vi "Configure Transducer.vi"(0 "VISA resource name":refnum<visa-resource-name>, 1 "Thermocouple Type (0: J)":i32(ring) items=["J", "K", "T", "E", "N", "R"], 2 "Enable Thermocouple Check (F: Disable)":bool, 3 "Reference Junction Temperature (0 Degrees C)":dbl, 5 "Enable Offset Compensation (F: Disable)":bool, 7 "Enable RTD Power Limit (F: Disable)":bool, 9 "Enable Thermistor Power Limit (F: Disable)":bool, 11 "error in (no error)":errorcluster, 12 "Reference Junction Temperature Adjust (0 Degrees C)":dbl, 13 "Thermocouple Reference Junction Type (0: Internal)":i32(ring) items=["Internal", "Fixed"]) -> (4 "VISA resource name out":refnum<visa-resource-name>, 15 "error out":errorcluster)   [LabVIEW 2013, in "Agilent 3446X Series.lvlib"]
doc: "Configures the transducer settings. Supplements \"Configure Temperature\". All of these options apply only to the 34465A and 34470A."
uses:
  <instrlib>/Agilent 3446X Series/Agilent 3446X Series.lvlib
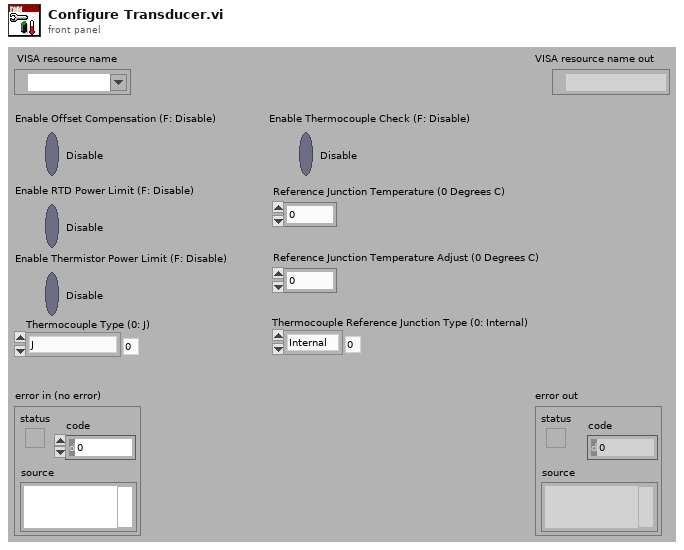
[diagram p1: front panel]
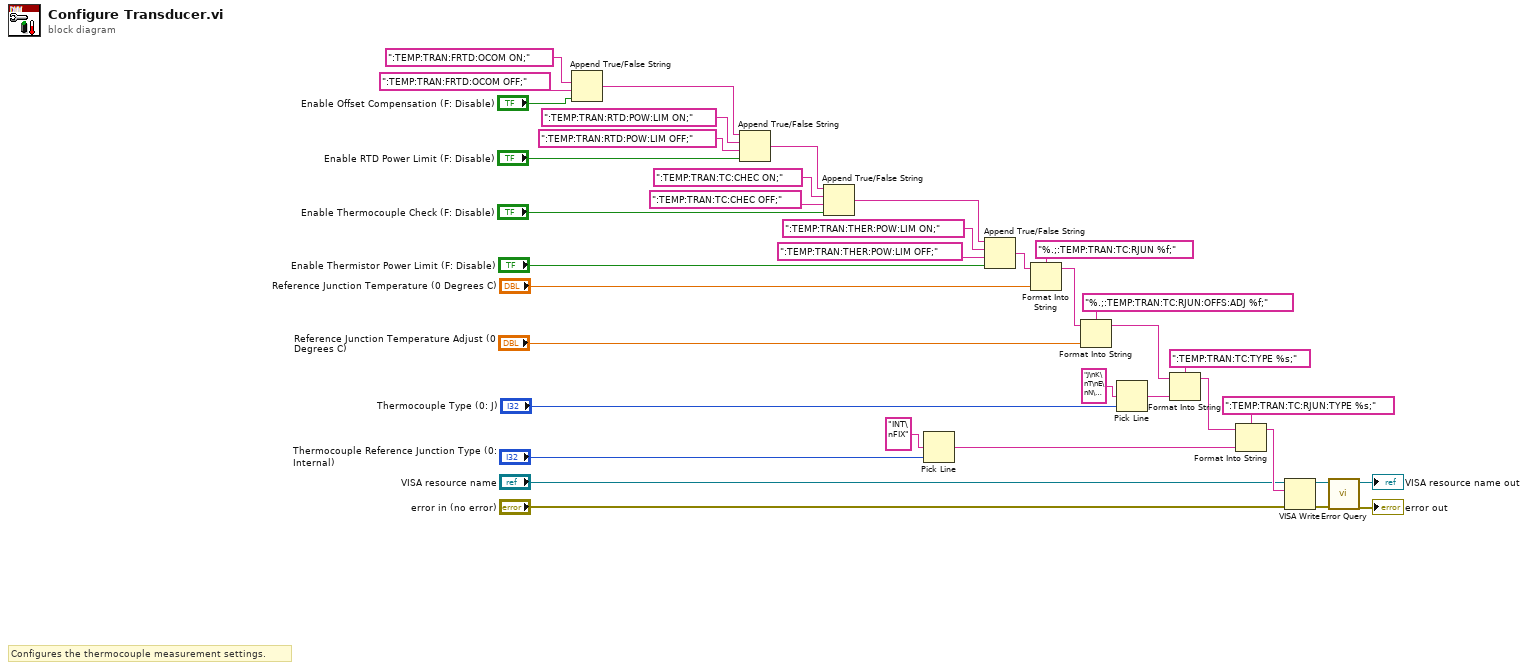
[diagram p0: block diagram]
diagram:
  # "Configures the thermocouple measurement settings."
  n1 = Append True/False String(1:"Enable Offset Compensation (F: Disable)", 2:":TEMP:TRAN:FRTD:OCOM OFF;" ("false string"), 3:":TEMP:TRAN:FRTD:OCOM ON;" ("true string")) -> (0:w21:string)  [unwired: 1 in]
  n2 = Append True/False String(1:"Enable RTD Power Limit (F: Disable)", 2:":TEMP:TRAN:RTD:POW:LIM OFF;" ("false string"), 3:":TEMP:TRAN:RTD:POW:LIM ON;" ("true string"), 4:w21) -> (0:w18:string)
  n3 = Append True/False String(1:"Enable Thermocouple Check (F: Disable)", 2:":TEMP:TRAN:TC:CHEC OFF;" ("false string"), 3:":TEMP:TRAN:TC:CHEC ON;" ("true string"), 4:w18) -> (0:w15:string)
  n4 = Pick Line(multi-line string="INT\nFIX", line index="Thermocouple Reference Junction Type (0: Internal)") -> (output string=w3:string)  [unwired: 1 in]
  n5 = Append True/False String(1:"Enable Thermistor Power Limit (F: Disable)", 2:":TEMP:TRAN:THER:POW:LIM OFF;" ("false string"), 3:":TEMP:TRAN:THER:POW:LIM ON;" ("true string"), 4:w15) -> (0:w14:string)
  n6 = Format Into String(format string="%.;:TEMP:TRAN:TC:RJUN %f;", initial string=w14, "Reference Junction Temperature (0 Degrees C)") -> (resulting string=w11:string)  [unwired: 1 in, 1 out]
  n7 = Format Into String(format string="%.;:TEMP:TRAN:TC:RJUN:OFFS:ADJ %f;", initial string=w11, "Reference Junction Temperature Adjust (0 Degrees C)") -> (resulting string=w7:string)  [unwired: 1 in, 1 out]
  n8 = Pick Line(multi-line string="J\nK\nT\nE\nN\nR", line index="Thermocouple Type (0: J)") -> (output string=w6:string)  [unwired: 1 in]
  n9 = Format Into String(format string=":TEMP:TRAN:TC:TYPE %s;", initial string=w7, w6) -> (resulting string=w4:string)  [unwired: 1 in, 1 out]
  n10 = Format Into String(format string=":TEMP:TRAN:TC:RJUN:TYPE %s;", initial string=w4, w3) -> (resulting string=w26:string)  [unwired: 1 in, 1 out]
  n11 = VISA Write(VISA resource name="VISA resource name", write buffer=w26, error in (no error)="error in (no error)") -> (VISA resource name out=w38:refnum<visa-resource-name>, error out=w37:errorcluster)  [unwired: 1 out]
  n12 = call <instrlib>:"Error Query.vi"("error in (no error)"=w37, "VISA resource name"=w38) -> ("error out"=→"error out":errorcluster, "VISA resource name out"=→"VISA resource name out":refnum<visa-resource-name>)  [unwired: 8 out]
